vi "SetMultiColColor.vi"(7 "色指定":cluster{"背景色":u32, "文字色":u32}, 8 "Error In":errorcluster caption="エラー入力", 9 "長さ":i32, 10 "開始列":i32, 11 "Tbl refnum":refnum<vi>) -> (0 "Error Out":errorcluster caption="エラー出力", 3 "Tbl refnum出力":refnum<vi>)   [LabVIEW 2014]
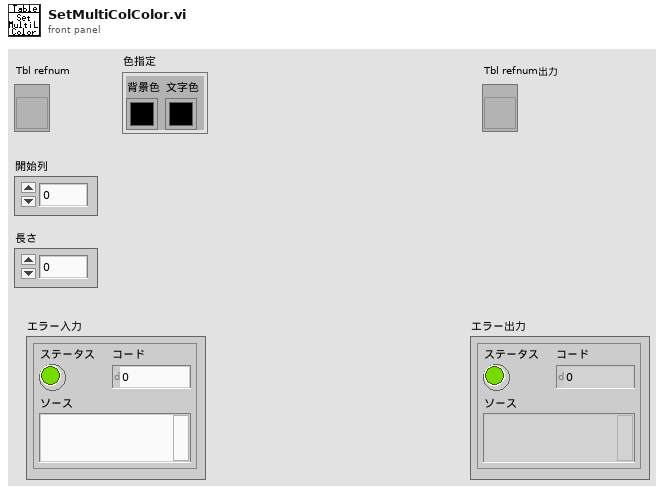
[diagram p1: front panel]
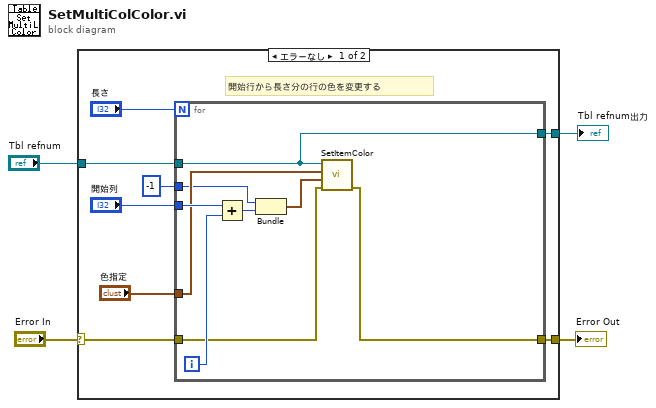
[diagram p0: block diagram]
diagram:
  n1 = case shown="エラーなし" "Error In" {
    selector: "Error In" -> [w8 w23]
    tunnel: [w7 w23] -> w3
    tunnel: "Tbl refnum" -> [w6 w22]
    tunnel: [w5 w22] -> w1
    frame No Error {
      # "開始行から長さ分の行の色を変更する"
      n2 = for {
        N: "長さ" -> [_]
        tunnel: w6 -> [w15]
        tunnel: "開始列" -> [w21]
        tunnel: -1 -> [w13]
        tunnel: "色指定" -> [w18]
        tunnel: w8 -> [w17]
        tunnel: [w16] -> w7
        tunnel: [w15] -> w5
        i -> [w20]
        n3 = Add(x=w21, y=w20) -> (x+y=w14:i32)
        n4 = Bundle(w13, w14) -> (w19:cluster{i32, i32})  [unwired: 1 in]
        n5 = call "SetItemColor.vi"("エラー入力(エラーなし)"=w17, "行列指定"=w19, "色指定"=w18, "Tbl refnum"=w15) -> ("エラー出力"=w16:errorcluster)  [unwired: 7 in]
      }
    }
    frame Error {
    }
  }
  "Error Out" <- w3
  "Tbl refnum出力" <- w1
